vi "DAQ Test.vi"(7 "rate":dbl=1000.0, 10 "data":dynamicdata(waveform), 11 "device name":tag="cDAQ2Mod1") -> (2 "error out":errorcluster, 3 "task out":refnum<k21>)   [LabVIEW 2019]
uses:
  <vilib>/DAQmx/write.llb/DAQmx Write (Analog 1D Wfm NChan NSamp).vi
  <vilib>/DAQmx/create/channels.llb/DAQmx Create Channel (AO-Voltage-Basic).vi
  <vilib>/DAQmx/configure/timing.llb/DAQmx Timing (Sample Clock).vi
  <vilib>/DAQmx/miscellaneous.llb/DAQmx Fill In Error Info.vi
  GBV_Ref.vi
  <resource>/objmgr/daqmx.rc
panel:
  in  "error in":errorcluster
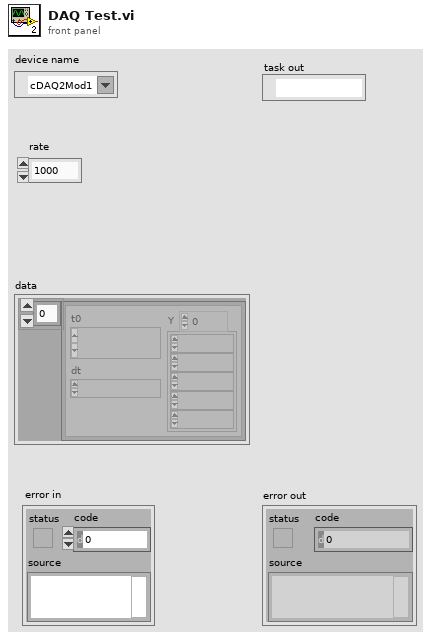
[diagram p1: front panel]
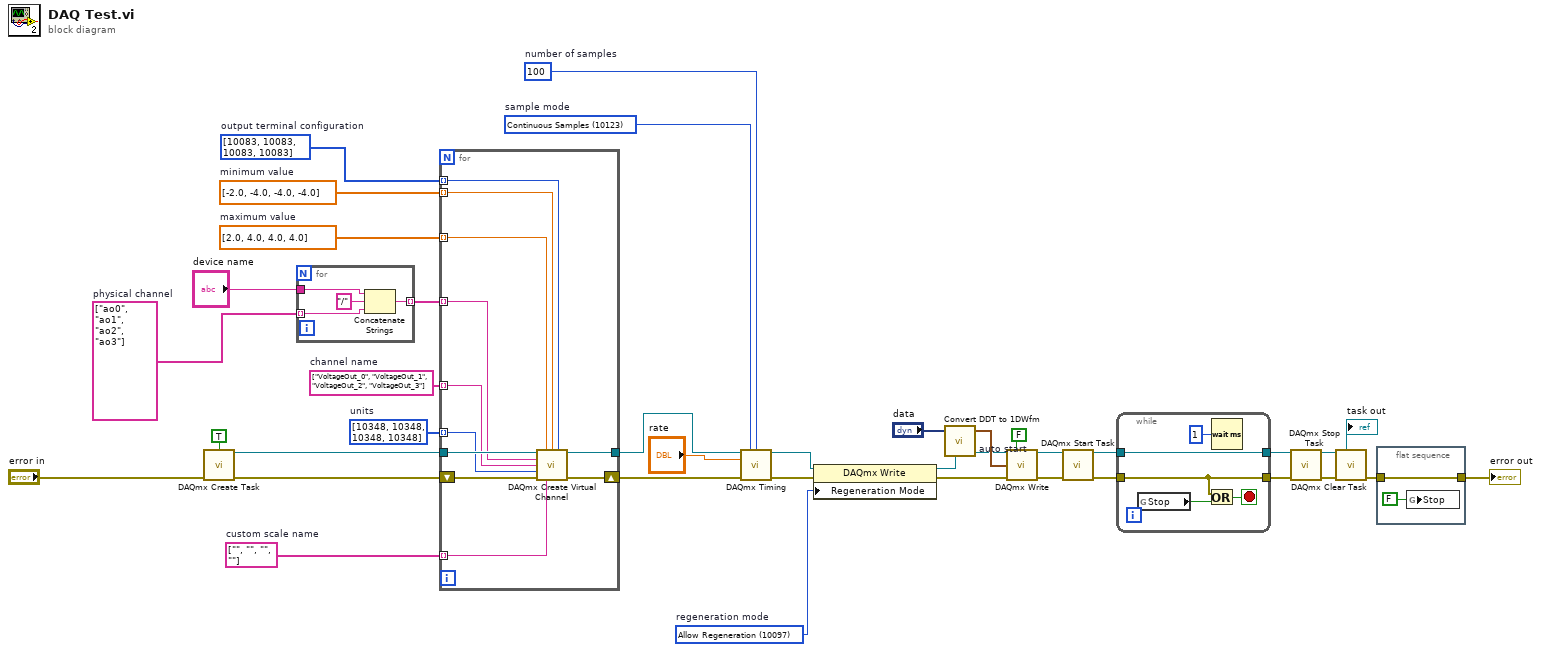
[diagram p0: block diagram]
diagram:
  w13 = FALSE  # auto start
  w18 = 10097 items=["Allow Regeneration"=10097, "Do Not Allow Regeneration"=10158]  # regeneration mode
  w21 = 10123 items=["Finite Samples"=10178, "Continuous Samples"=10123, "Hardware Timed Single Point"=12522]  # sample mode
  w23 = 100  # number of samples
  w26 = i32[] [10083, 10083, 10083, 10083] items=["Default"=-1, "RSE"=10083, "Differential"=10106, "Pseudodifferential"=12529]  # output terminal configuration
  w27 = string[] ["", "", "", ""]  # custom scale name
  w28 = i32[] [10348, 10348, 10348, 10348] items=["Volts"=10348, "From Custom Scale"=10065]  # units
  w29 = string[] ["VoltageOut_0", "VoltageOut_1", "VoltageOut_2", "VoltageOut_3"]  # channel name
  w31 = dbl[] [2.0, 4.0, 4.0, 4.0]  # maximum value
  w32 = dbl[] [-2.0, -4.0, -4.0, -4.0]  # minimum value
  w35 = string[] ["ao0", "ao1", "ao2", "ao3"]  # physical channel
  n1 = call <vilib>:"DAQmx Create Task.vi"("auto cleanup"=TRUE, "error in"="error in") -> ("task out"=w34:refnum<k21>, "error out"=w33:errorcluster)  [unwired: 12 in]
  n2 = for {
    tunnel: [w40] -> w30 mode=indexing
    tunnel: "device name" -> [w39]
    tunnel: w35 -> [w37] mode=indexing
    n3 = Concatenate Strings(w39, "/" ("string"), w37) -> (w40:string)
  }
  n4 = for {
    tunnel: w34 -> [w51]
    tunnel: [w49] -> w25
    tunnel: w32 -> [w47] mode=indexing
    tunnel: w31 -> [w46] mode=indexing
    tunnel: w30 -> [w45] mode=indexing
    tunnel: w29 -> [w44] mode=indexing
    tunnel: w28 -> [w43] mode=indexing
    tunnel: w27 -> [w42] mode=indexing
    shift-right: [w48] -> w24
    shift-left: w33 -> [w50]
    tunnel: w26 -> [w41] mode=indexing
    n5 = call-poly <vilib>:"DAQmx Create Virtual Channel.vi"("task in"=w51, "maximum value"=w46, "minimum value"=w47, "output terminal configuration"=w41, "physical channels"=w45, "name to assign"=w44, "units"=w43, "error in"=w50, "custom scale name"=w42) -> ("task out"=w49:refnum<k21>, "error out"=w48:errorcluster)  [unwired: 5 in]
  }
  n6 = call-poly <vilib>:"DAQmx Timing.vi"("task/channels in"=w25, "sample mode"=w21, "samples per channel"=w23, "rate"="rate", "error in"=w24) -> ("task out"=w20:refnum<k21>, "error out"=w19:errorcluster)  [unwired: 9 in]
  n7 = property class="DAQmx Write"(reference=w20, error in=w19, "Regeneration Mode"=w18) -> (reference out=w9:refnum<k21>, error out=w10:errorcluster)
  n8 = call <vilib>:"Convert DDT to 1DWfm.vi"("Dynamic Data Type"="data") -> ("Array of Waveforms"=w15:waveform(dbl)[])  [unwired: 3 in]
  n9 = call-poly <vilib>:"DAQmx Write.vi"("task/channels in"=w9, "auto start"=w13, "data"=w15, "error in"=w10) -> ("task out"=w11:refnum<k21>, "error out"=w12:errorcluster)  [unwired: 9 in, 1 out]
  n10 = call <vilib>:"DAQmx Start Task.vi"("task/channels in"=w11, "error in"=w12) -> ("task out"=w8:refnum<k21>, "error out"=w6:errorcluster)  [unwired: 12 in]
  n11 = while {
    tunnel: w8 -> [w56]
    tunnel: [w56] -> w7
    tunnel: w6 -> [w54]
    tunnel: [w54] -> w5
    stop <- w55 stop-if-true
    n12 = global read "GBV_Ref.vi" "Stop"() -> (w53:bool)
    n13 = Or(x=w54, y=w53) -> (x .or. y?=w55:bool)
    n14 = Wait (ms)(milliseconds to wait=u32 1) -> ()  [unwired: 1 out]
  }
  n15 = call <vilib>:"DAQmx Stop Task.vi"("task/channels in"=w7, "error in"=w5) -> ("task out"=w4:refnum<k21>, "error out"=w17:errorcluster)  [unwired: 12 in]
  "task out" <- w4
  n16 = call <vilib>:"DAQmx Clear Task.vi"("task in"=w4, "error in"=w17) -> ("error out"=w3:errorcluster)  [unwired: 13 in]
  n17 = flat-sequence {
    tunnel: w3 -> [w58]
    tunnel: [w58] -> w2
    frame #0 {
      n18 = global write "GBV_Ref.vi" "Stop"(FALSE ("Stop")) -> ()
    }
  }
  "error out" <- w2
